vi "New Element.vi"(8 "error in (no error)":errorcluster, 10 "Element":variant, 11 "CircularBuffer":refnum<class "CircularBuffer.lvclass">) -> (0 "error out":errorcluster, 2 "newElementIndex":i32=1, 3 "CircularBuffer out":refnum<class "CircularBuffer.lvclass">)   [LabVIEW 2013, in "CircularBuffer.lvclass"]
doc: "---------------------------------------------------------------\nJKI State Machine Objects™\nhttp://jki.net/state-machine-objects/\nCopyright (C) 2005-2015, JKI <info@jki.net>\nALL RIGHTS RESERVEDJKI State Machine Objects (SMO) 1.0.0.4\nJKI - JKI\nCopyright (c) 2015, JKI"
uses:
  CircularBuffer.lvclass
  types/type/type.lvclass
panel:
  # "For instructions on how to use the JKI State Machine Objects, examples and video tutorials, visit:\nhttp://jki.net/state-machine-objects/\n\nJKI State Machine Objects™\nhttp://jki.net/state-machine-objects/\nCopyright (C) 2005-2015, JKI <info@jki.net>\nALL RIGHTS RESERVED"
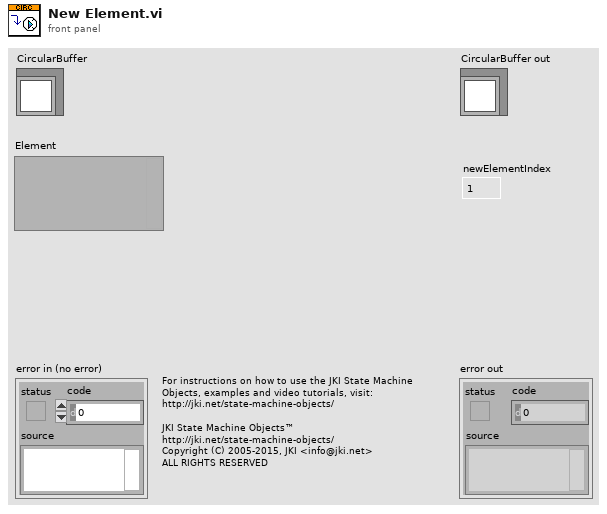
[diagram p1: front panel]
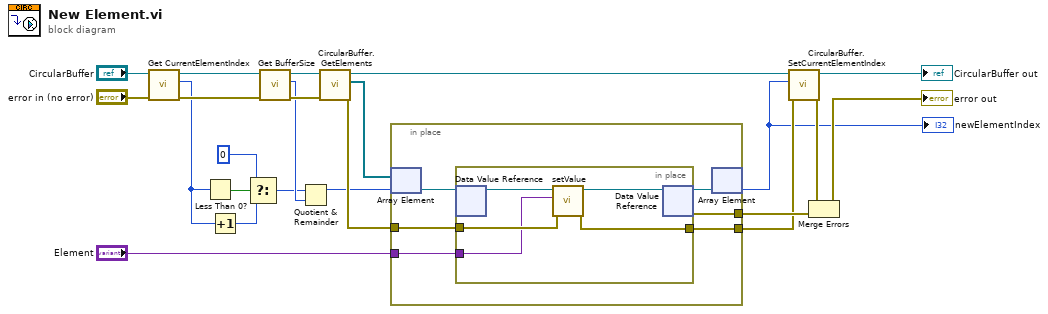
[diagram p0: block diagram]
diagram:
  n1 = call "Get CurrentElementIndex.vi"("error in (no error)"="error in (no error)", "CircularBuffer"="CircularBuffer") -> ("error out"=w15:errorcluster, "Current Element index"=w7:i32, "CircularBuffer out"=w17:refnum<class "CircularBuffer.lvclass">)  [unwired: 7 in]
  n2 = Less Than 0?(x=w7) -> (x < 0?=w9:bool)
  n3 = Increment(x=w7) -> (x+1=w5:i32)
  n4 = Select(t=0, s=w9, f=w5) -> (s? t:f=w6:i32)
  n5 = call "Get BufferSize.vi"("error in (no error)"=w15, "CircularBuffer"=w17) -> ("error out"=w14:errorcluster, "BufferSize"=w13:i32, "CircularBuffer out"=w16:refnum<class "CircularBuffer.lvclass">)  [unwired: 7 in]
  n6 = Quotient & Remainder(x=w6, y=w13) -> (x-y*floor(x/y)=w2:i32)  [unwired: 1 out]
  n7 = call "CircularBuffer.GetElements.vi"("error in (no error)"=w14, "CircularBuffer in"=w16) -> ("error out"=w22:errorcluster, "Elements"=w10:refnum<data-value>[], "CircularBuffer out"=w12:refnum<class "CircularBuffer.lvclass">)  [unwired: 7 in]
  n8 = in-place {
    in-place-border: w22 -> [w29]
    in-place-border: [w28] -> w4
    in-place-border: [w27] -> w21
    in-place-border: "Element" -> [w26]
    n9 = in-place-array #1(w10, w2) -> (w25:refnum<data-value>)
    n10 = in-place {
      in-place-border: w29 -> [w32]
      in-place-border: [w31] -> w28
      in-place-border: w26 -> [w30]
      n11 = in-place-dvr #2(w25) -> (w34:refnum<class "type.lvclass">)  [unwired: 1 out]
      n12 = call-dynamic "setValue.vi"("error in (no error)"=w32, "value"=w30, "type in"=w34) -> ("error out"=w31:errorcluster, "type out"=w33:refnum<class "type.lvclass">)  [unwired: 7 in]
      n13 = in-place-dvr #2(w33) -> (w24:refnum<data-value>, w27:errorcluster)
    }
    n14 = in-place-array #1(w24) -> (w1:i32)  [unwired: 1 out]
  }
  "newElementIndex" <- w1
  n15 = call "CircularBuffer.SetCurrentElementIndex.vi"("error in (no error)"=w4, "Index"=w1, "CircularBuffer"=w12) -> ("error out"=w3:errorcluster, "CircularBuffer out"=→"CircularBuffer out":refnum<class "CircularBuffer.lvclass">)  [unwired: 7 in]
  n16 = Merge Errors(w3, w21) -> (→"error out":errorcluster)
